vi "test3Dgraph.vi"() -> ()   [LabVIEW 2014]
uses:
  <vilib>/Math Plots/3D Math Plots/3D Surface/3D Surface Datatype/3D Surface Datatype.lvclass
  <vilib>/Math Plots/3D Math Plots/3D Surface/3D Surface Datatype/Public/Plot Helper (Vector).vi
  <vilib>/Math Plots/3D Math Plots/3D Surface/3D Surface XCtrl/3D Surface.xctl
  <vilib>/Analysis/Matrix/Datatypes/RealMatrix.ctl
  <vilib>/Analysis/Matrix/NI_Matrix.lvlib
panel:
  out "output array":dbl[](array[numeric])
  out "subarray":T1
  in  "length 2":i32
  in  "index 2":i32
  in  "length":i32
  in  "index":i32
  out "output matrix":T1
  out "3D Surface":refnum<class "3D Plot Datatype.lvclass">[](xcontrol)
  out "appended array":dbl[][](array[numeric])
  out "Y":dbl[](array[numeric])
  out "X":dbl[](array[numeric])
  out "Z":dbl[][](array[numeric])
  in  "Max":dbl format="%#_13g"
  in  "Step":dbl format="%#_13g"
  in  "Init Value":dbl format="%#_13g"
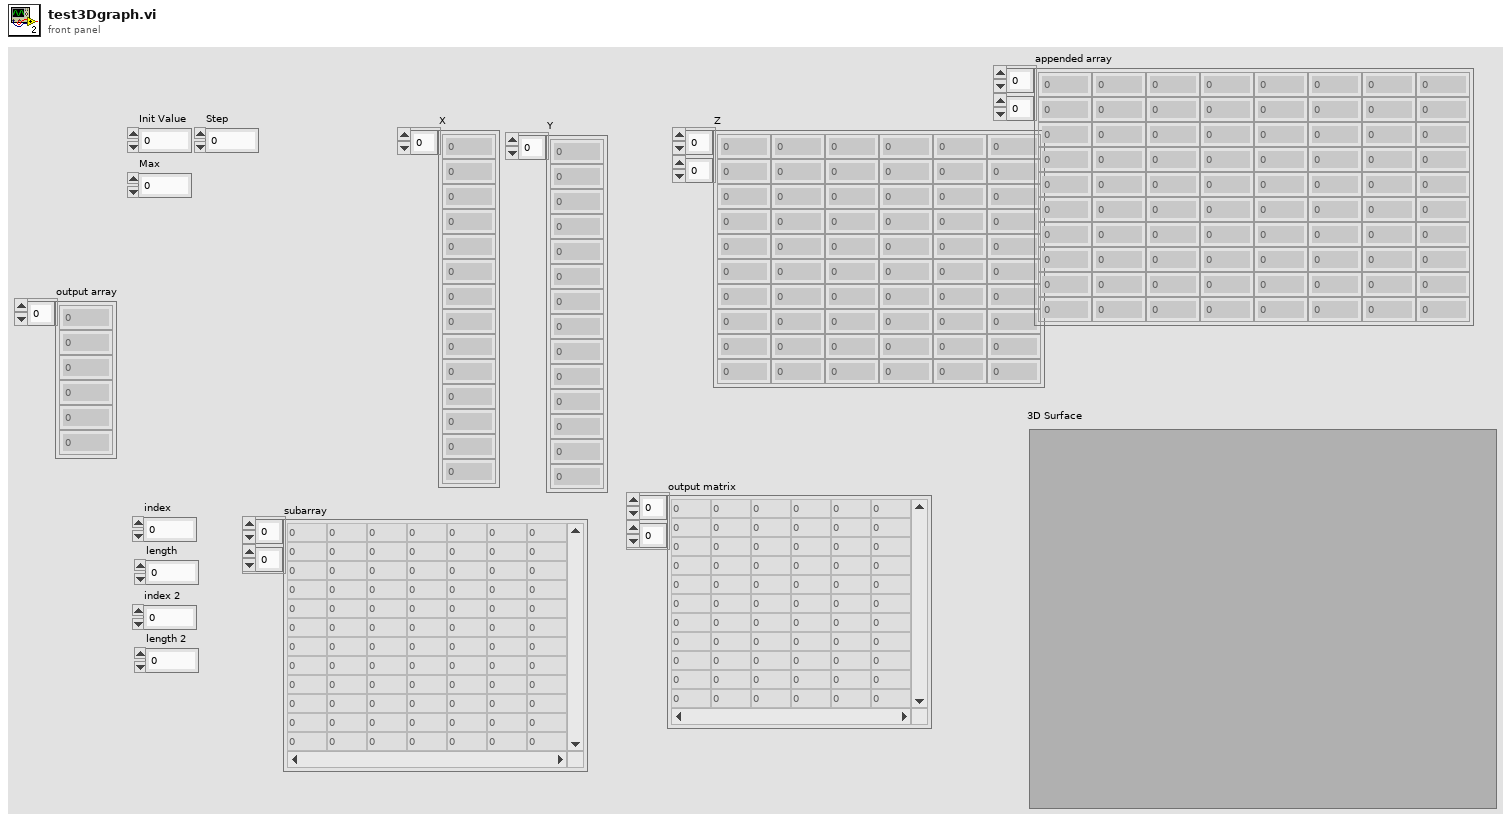
[diagram p1: front panel]
types:
  T1 = typedef "NI_Matrix.lvlib/RealMatrix.ctl" = dbl[][]
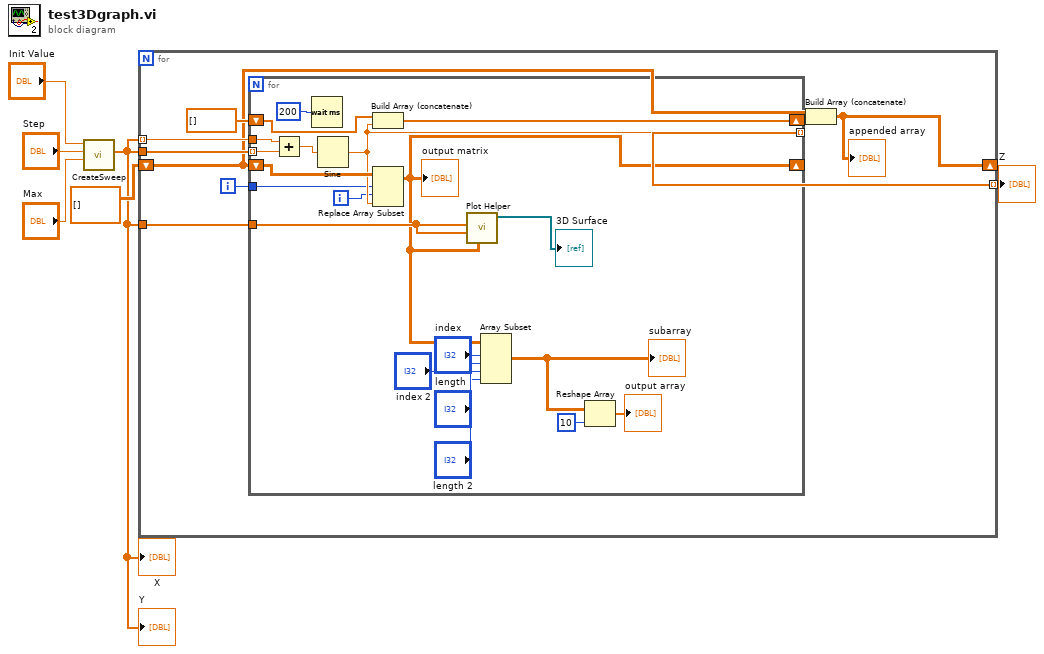
[diagram p0: block diagram]
diagram:
  n1 = call "CreateSweep.vi"("Max"="Max", "Step"="Step", "Init Value"="Init Value") -> ("Array"=w1:dbl[])  [unwired: 8 in]
  "X" <- w1
  "Y" <- w1
  n2 = for {
    tunnel: w1 -> [w15] mode=indexing
    tunnel: w1 -> [w11]
    tunnel: [w14] -> w2 mode=indexing
    shift-right: [w10] -> _
    shift-left: dbl[][] [] -> [w9]
    tunnel: w1 -> [w7]
    i -> [w8]
    n3 = for {
      tunnel: w11 -> [w34] mode=indexing
      tunnel: w15 -> [w35]
      tunnel: [w28] -> w14 mode=indexing
      shift-right: [w31] -> w12
      shift-left: dbl[] [] -> [w32]
      tunnel: w8 -> [w27]
      tunnel: w7 -> [w24]
      shift-right: [w23] -> _
      shift-left: w9 -> [w29]
      i -> [w26]
      n4 = Add(x=w35, y=w34) -> (x+y=w33:dbl)
      n5 = Wait (ms)(milliseconds to wait=u32 200) -> ()  [unwired: 1 out]
      n6 = Sine(x=w33) -> (sin(x)=w28:dbl)
      n7 = Build Array (concatenate)(w32, w28) -> (w31:dbl[])
      n8 = Replace Array Subset(array=w29, new element=w28, index (row)=w27, index (col)=w26) -> (w23:T1)
      "output matrix" <- w23
      n9 = call-poly <vilib>:"Plot Helper.vi"("z matrix"=w23, "y vector"=w24, "x vector"=w24) -> ("3D Plot lvclass Array out"=→"3D Surface":refnum<class "3D Plot Datatype.lvclass">[])  [unwired: 3 in, 5 out]
      n10 = Array Subset(array=w23, index (row)="index", length (row)="length", index (col)="index 2", length (col)="length 2") -> (w18:T1)
      "subarray" <- w18
      n11 = Reshape Array(w18, 10 ("dimension size")) -> (→"output array":dbl[])
    }
    n12 = Build Array (concatenate)(w9, w12) -> (w10:dbl[][])
    "appended array" <- w10
  }
  "Z" <- w2
